vi "ex2.vi"() -> ()   [LabVIEW 2015]
panel:
  out "Specific Harmonic":i32[](array[numeric])
  out "THD":i32
  out "Current RMS":dbl format="%#_13g"
  out "Voltage RMS":dbl format="%#_13g"
  out "data":dynamicdata(graph)
  in  "stop":bool
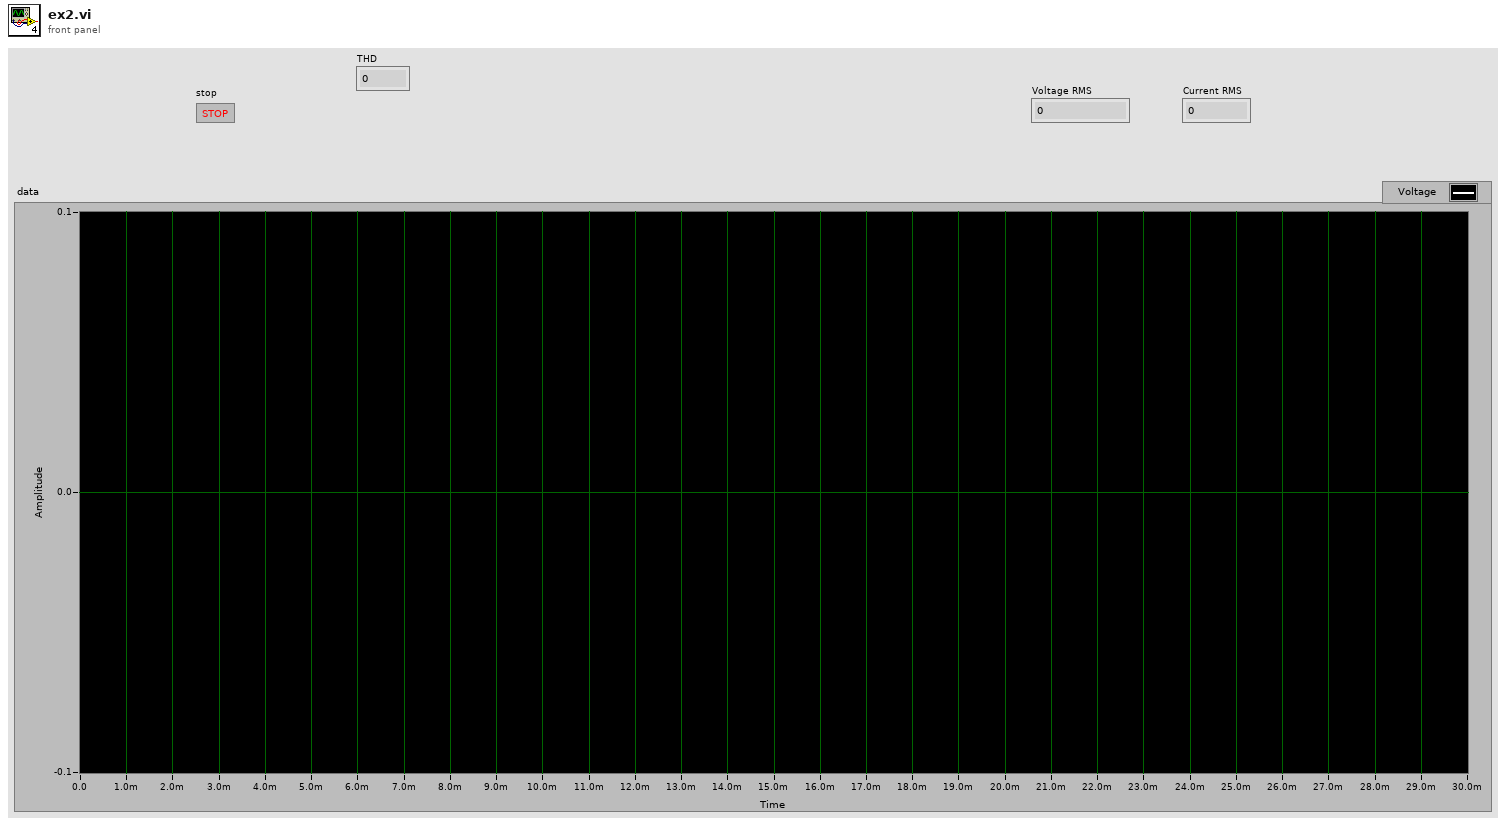
[diagram p1: front panel]
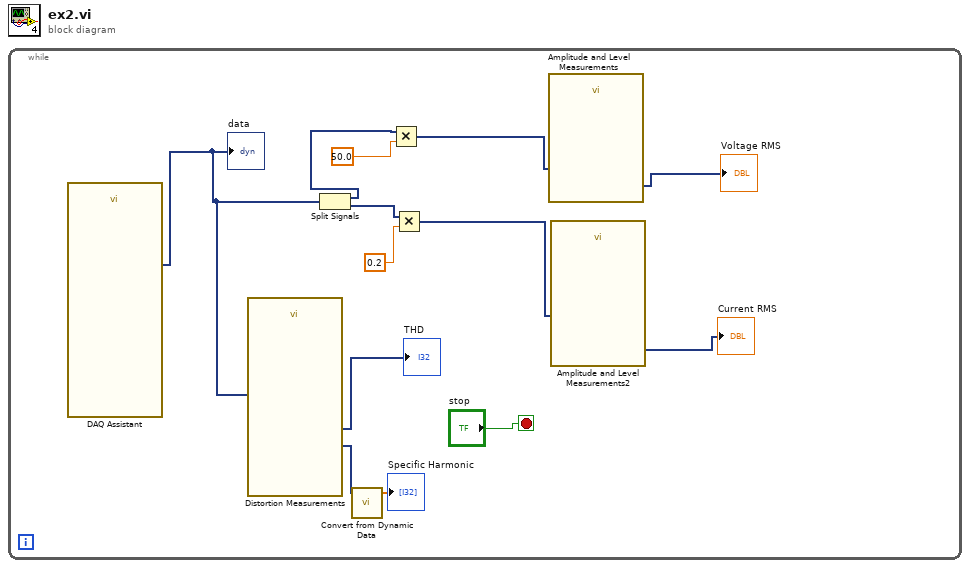
[diagram p0: block diagram]
diagram:
  n1 = while {
    stop <- "stop" stop-if-true
    n2 = call "DAQ Assistant"() -> ("data"=w1:dynamicdata)  [unwired: 16 in, 3 out]
    "data" <- w1
    n3 = call "Distortion Measurements"("Signals"=w1) -> ("Specific Harmonic"=w3:dynamicdata, "THD"=→"THD":dynamicdata)  [unwired: 7 in, 2 out]
    n4 = Split Signals(w1) -> (w10:dynamicdata, w9:dynamicdata)  [unwired: 2 in]
    n5 = call "Convert from Dynamic Data"("Dynamic Data Type"=w3) -> ("Array"=→"Specific Harmonic":dbl[])  [unwired: 3 in]
    n6 = Multiply(x=w10, y=50.0) -> (x*y=w8:dynamicdata)
    n7 = Multiply(x=w9, y=0.2) -> (x*y=w7:dynamicdata)
    n8 = call "Amplitude and Level Measurements"("Signals"=w8) -> ("Cycle RMS"=→"Voltage RMS":dynamicdata)  [unwired: 13 in, 1 out]
    n9 = call "Amplitude and Level Measurements2"("Signals"=w7) -> ("Cycle RMS"=→"Current RMS":dynamicdata)  [unwired: 12 in, 2 out]
  }
